vi "Write Event.vi"(8 "error in (no error)":errorcluster, 10 "Event.lvclass":refnum<class "Event.lvclass">, 11 "EventLog in":refnum<class "EventLog.lvclass">) -> (0 "error out":errorcluster, 3 "EventLog out":refnum<class "EventLog.lvclass">)   [LabVIEW 2019, in "EventLog.lvlib" / "EventLog.lvclass"]
uses:
  EventLog.lvclass
  Classes/Event/Event.lvclass
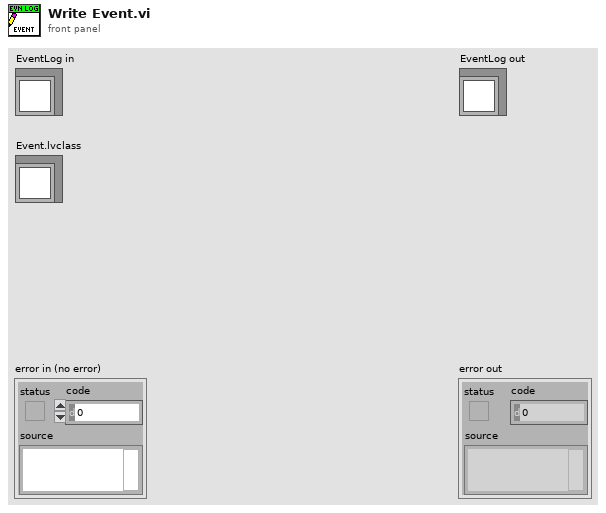
[diagram p1: front panel]
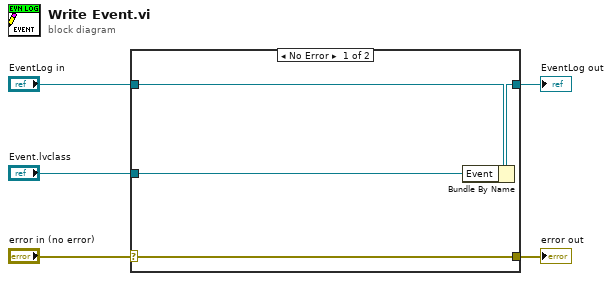
[diagram p0: block diagram]
diagram:
  n1 = case shown="No Error" "error in (no error)" {
    selector: "error in (no error)" -> [w9 w10]
    tunnel: [w9 w10] -> w4
    tunnel: [w7 w11] -> w2
    tunnel: "EventLog in" -> [w8 w11]
    tunnel: "Event.lvclass" -> [w6 _]
    frame No Error {
      n2 = Bundle By Name(cluster=w8, "Event"=w6) -> (w7:refnum<class "EventLog.lvclass">)
    }
    frame Error {
    }
  }
  "error out" <- w4
  "EventLog out" <- w2
